vi "CSM - Get New State Notifier Event.vi"(8 "Error In":errorcluster caption="error in (no error)", 11 "Name (\"\" to Use UUID)":string) -> (0 "error out":errorcluster, 3 "New State Notifier Event":refnum<user-event>)   [LabVIEW 2017, in "Communicable State Machine.lvlib"]
doc: "Obtains a user event refnum, which is suitable for CSM modules containing an Event Structure. CSM modules with an Event Structure typically wait at the Event Structure. The user event refnum this VI obtains is used to interrupt the wait in the Event Structure when a new message is received, allowing the module to continue execution.\n\n-- <b>Controls</b> --\n\n- <b>Name (\"\" to use UUID)</b>: CSM module name. Refer to *CSM Naming Rules* for module naming rules.\n\n-- <b>Indicators</b> --\n\n- <b>New State Notifier Event</b>: User event refnum, which is used to interrupt the CSM module's wait in the Event Structure when a message is received."
uses:
  Communicable State Machine.lvlib
  _Support/CSMQ/_CSMOFGVOPER.ctl
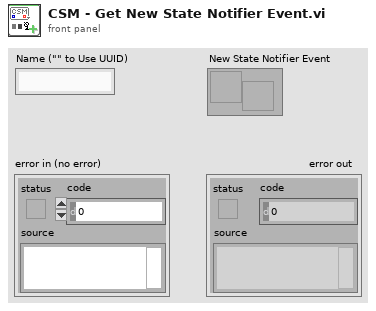
[diagram p1: front panel]
types:
  T1 = typedef "Communicable State Machine.lvlib/_CSMOFGVOPER.ctl" = enum16{"Create If not Exist", "Get By Name", "List", "Check If Name Exists", "Release", "Module Status", "Create Status Event Handler", "Destroy Status Event Handler", "Clear Invalid Objs"}
  T2 = typedef "Communicable State Machine.lvlib/_CSMObj.ctl" = cluster{"info":T3, "Refs":T5}
  T3 = typedef "Communicable State Machine.lvlib/_CSMObj-Info.ctl" = cluster{"Module Name":string, "Requested Name":string, "Group Name":string, "Mode":T4, "Allowed Messages":string[]}
  T4 = typedef "Communicable State Machine.lvlib/_CSM_MODE.ctl" = enum16{"Not Exist", "Stand Alone", "CSM", "Worker", "Worker Agent", "Chain Node", "Chain"}
  T5 = typedef "Communicable State Machine.lvlib/_CSMObj-Refs.ctl" = cluster{"WatchDogQ":refnum<queue>, "CSMDataDVR":refnum<data-value>, "Queue":T6, "GroupDataDVR":refnum<data-value>, "TagMap":refnum<data-value>, "ExitEvent":refnum<user-event>, "NewStateEvent":refnum<user-event>, "StatusEvent":refnum<user-event>, "InterruptEvent":refnum<user-event>}
  T6 = typedef "Communicable State Machine.lvlib/Priority Queue.ctl" = cluster{"HPriorityQ":refnum<queue>, "LowPriorityQ":refnum<queue>}
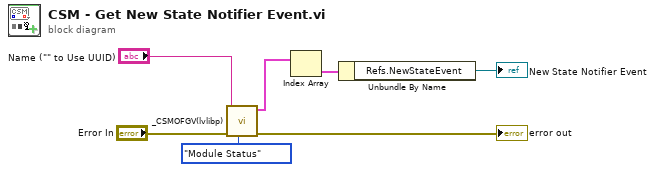
[diagram p0: block diagram]
diagram:
  n1 = call "_CSMOFGV(lvlibp).vi"("Operation"=_CSMOFGVOPER."Module Status", "Error In"="Error In", "Name (\"\" to Use UUID) In"="Name (\"\" to Use UUID)") -> ("error out"=→"error out":errorcluster, "Array"=w3:T2[])  [unwired: 6 in, 1 out]
  n2 = Index Array(array=w3) -> (element=w2:T2)  [unwired: 1 in]
  n3 = Unbundle By Name(w2) -> ("Refs.NewStateEvent"=→"New State Notifier Event":refnum<user-event>)
